vi "Go UP (Loaded).vi"(6 "Skip Loading?":bool, 7 "Model Name":T2, 8 "Error In":errorcluster, 9 "Intialize?":bool=TRUE, 10 "Inputs":T3) -> (0 "error out":errorcluster, 1 "Completed":bool, 3 "Results":T1, 4 "Status":cluster{"Status":string, "Elapsed Time":dbl}, 5 "Graph":dbl[][](array[numeric]))   [LabVIEW 2017]
doc: "Changelog:\n\n------------\nv0.1:\n- Bypass sensor 1 for all front\n\nv0.1:\n- Start Travel time taken from when the start moving command is given (previous state)\n- Total travel time is taken until the movement is stopped"
uses:
  controls/All Inputs.ctl
  controls/SACB DI.ctl
  controls/Model Name.ctl
  controls/Go UP (Loaded).ctl
  controls/FGV DO.ctl
panel:
  in  "Stall Time":u32=200
  out "Waveform Graph":dbl[][](graph)
  in  "Delay (for Rest)":u32=500
  in  "Timeout (ms)":u32=15000
  # "Inputs"
  # "Variables"
  # "Outputs"
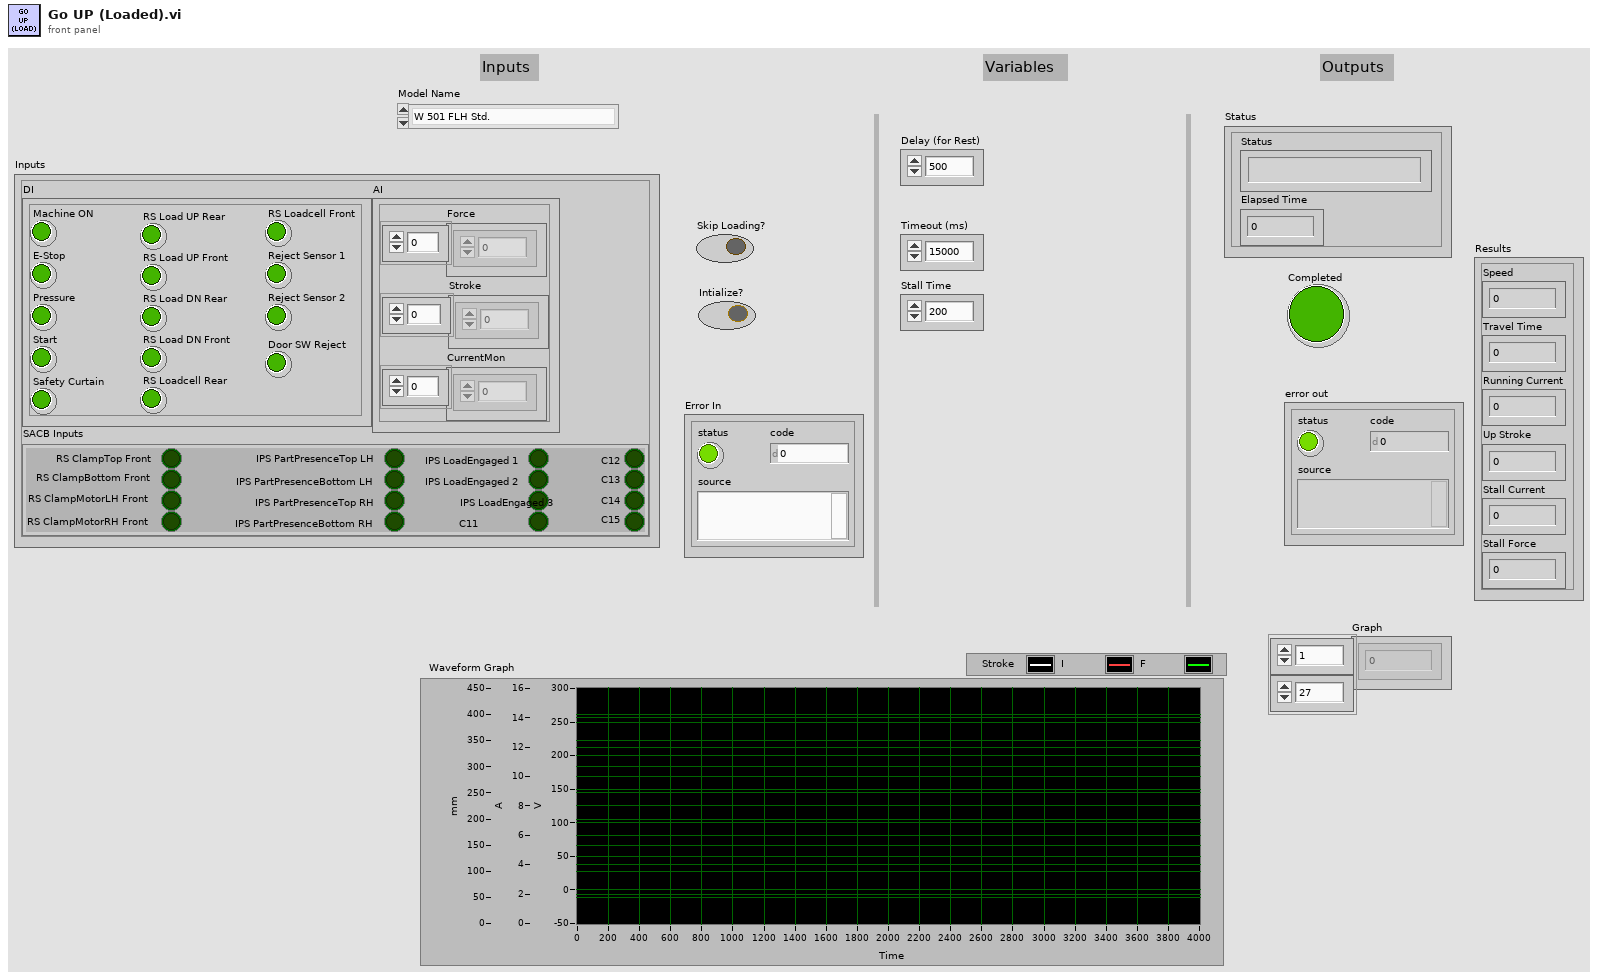
[diagram p1: front panel]
types:
  T1 = cluster{"Speed":dbl, "Travel Time":dbl, "Running Current":dbl, "Up Stroke":dbl, "Stall Current":dbl, "Stall Force":dbl}
  T2 = typedef "Model Name.ctl" = enum16{"W 501 FLH Std.", "W 501 FRH Std.", "W 601 FR RH Std", "W 601 FR LH Std", "W 601 RR RH Std", "W 601 RR LH Std", "W 601 FR RH AP", "W 601 FR LH AP", "W 601 RR RH AP", "W 601 RR LH AP"}
  T3 = typedef "All Inputs.ctl" = cluster{"DI":cluster{"Machine ON":bool, "E-Stop":bool, "Pressure":bool, "Start":bool, "Safety Curtain":bool, "RS Load UP Rear":bool, "RS Load UP Front":bool, "RS Load DN Rear":bool, "RS Load DN Front":bool, "RS Loadcell Rear":bool, "RS Loadcell Front":bool, "Reject Sensor 1":bool, "Reject Sensor 2":bool, "Door SW Reject":bool}, "AI":cluster{"Force":dbl[], "Stroke":dbl[], "CurrentMon":dbl[]}, "SACB Inputs":T4}
  T4 = typedef "SACB DI.ctl" = cluster{"RS ClampTop Front":bool, "RS ClampBottom Front":bool, "RS ClampMotorLH Front":bool, "RS ClampMotorRH Front":bool, "IPS PartPresenceTop LH":bool, "IPS PartPresenceBottom LH":bool, "IPS PartPresenceTop RH":bool, "IPS PartPresenceBottom RH":bool, "IPS LoadEngaged 1":bool, "IPS LoadEngaged 2":bool, "IPS LoadEngaged 3":bool, "C11":bool, "C12":bool, "C13":bool, "C14":bool, "C15":bool}
  T5 = typedef "Go UP (Loaded).ctl" = enum16{"Initialize", "Load UP Enable", "Check Bottom Position", "Go UP", "Wait for Stall", "Turn Off Supply", "Wait for Rest", "Done", "Error"}
  T6 = typedef "FGV DO.ctl" = enum16{"Initialize", "Start Task", "Clamping", "Load CYL", "Contactors", "Loadcell CYL", "BSL", "Read DO", "Clear Tasks", "Clear Task"}
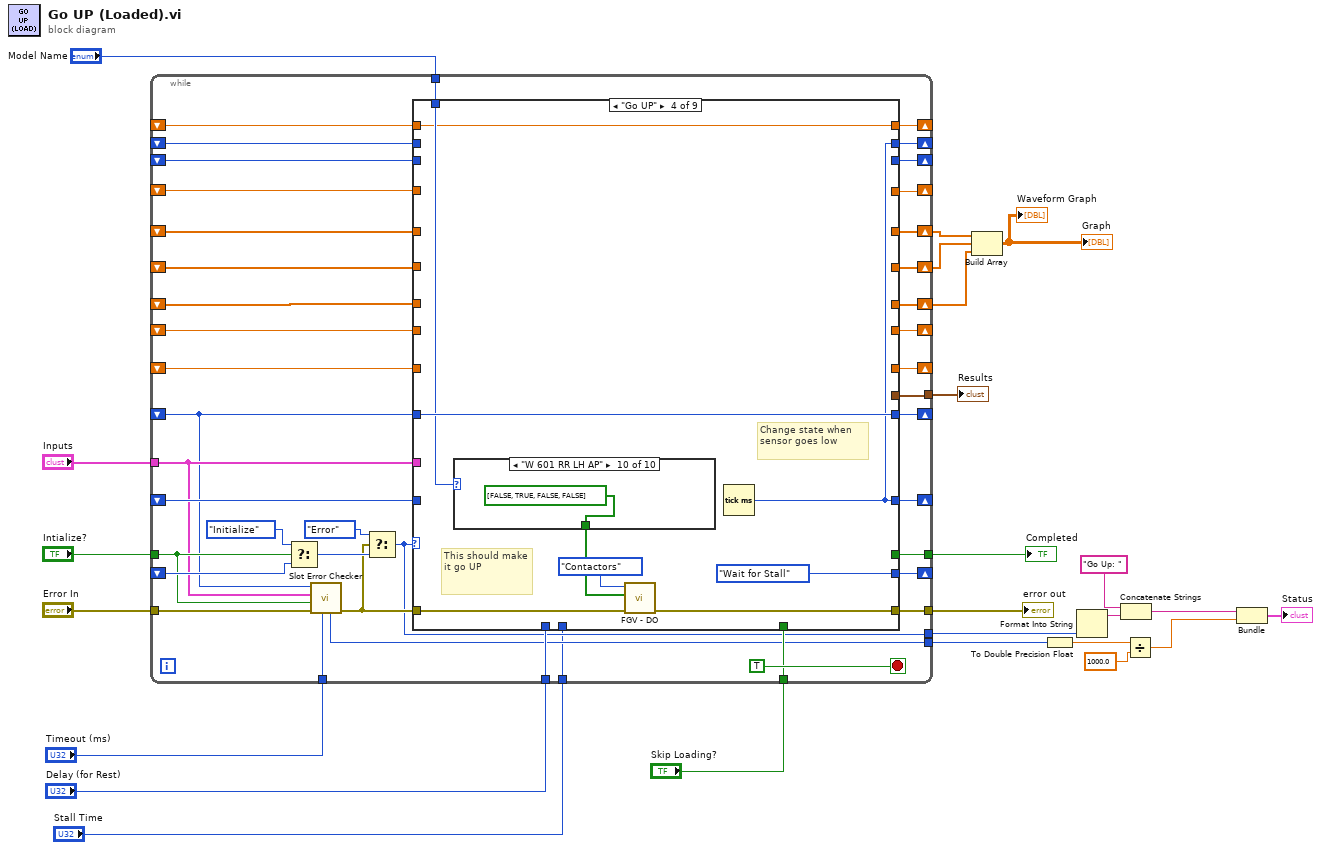
[diagram p0: block diagram]
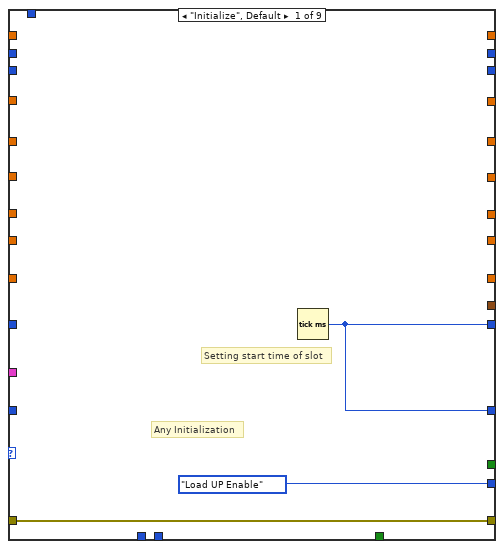
[diagram p2: hidden frame]
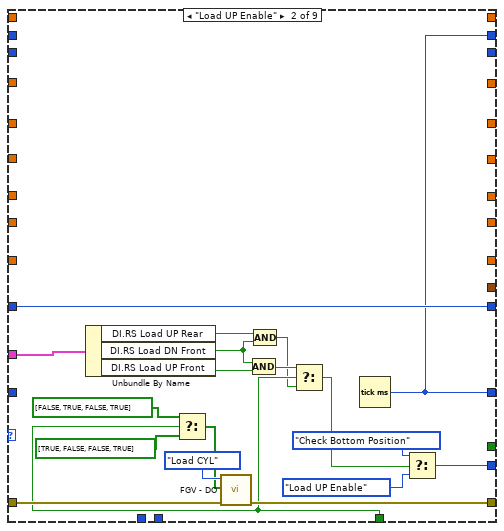
[diagram p3: hidden frame]
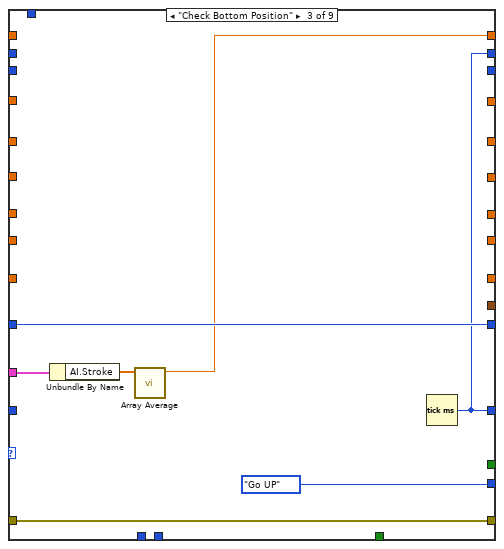
[diagram p4: hidden frame]
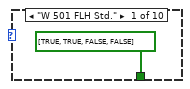
[diagram p5: hidden frame]
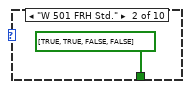
[diagram p6: hidden frame]
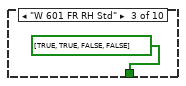
[diagram p7: hidden frame]
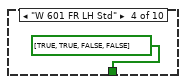
[diagram p8: hidden frame]
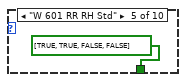
[diagram p9: hidden frame]
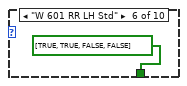
[diagram p10: hidden frame]
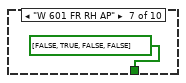
[diagram p11: hidden frame]
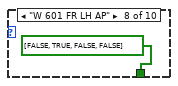
[diagram p12: hidden frame]
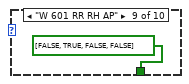
[diagram p13: hidden frame]
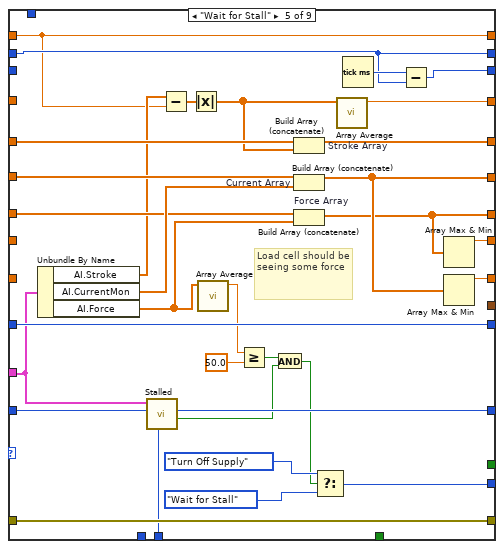
[diagram p14: hidden frame]
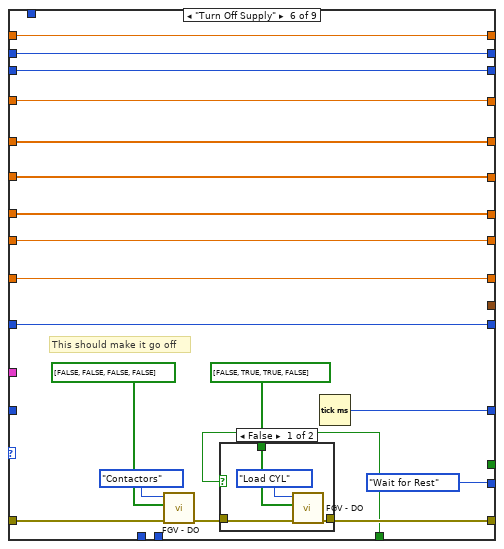
[diagram p15: hidden frame]
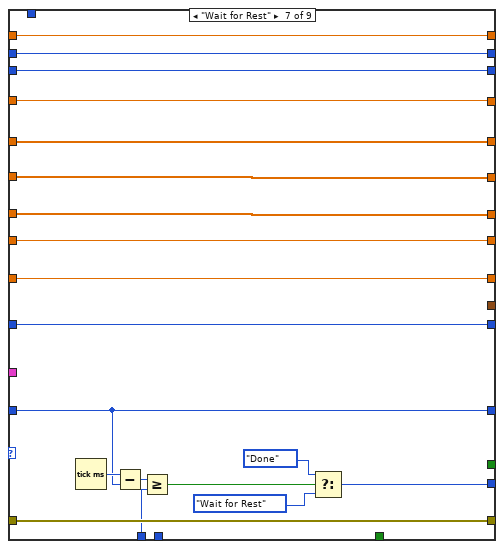
[diagram p17: hidden frame]
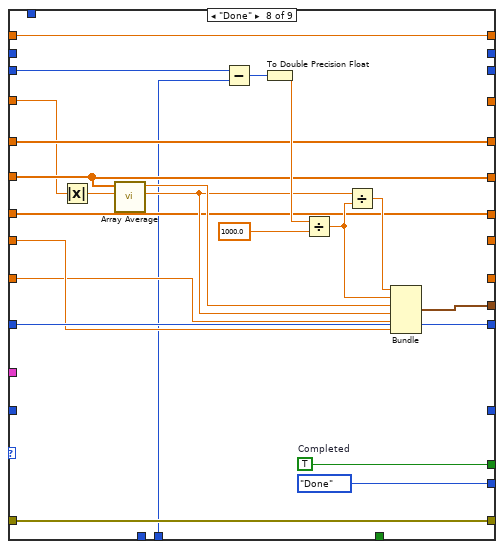
[diagram p18: hidden frame]
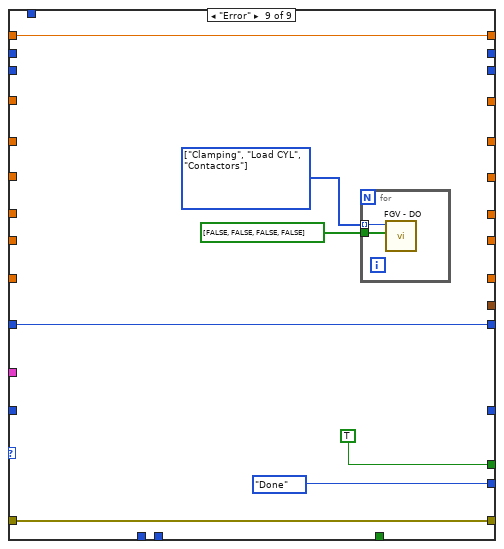
[diagram p19: hidden frame]
diagram:
  n1 = while {
    tunnel: "Intialize?" -> [w56]
    shift-right: [w63] -> _
    shift-left: _ -> [w65]
    shift-right: [w62] -> _
    shift-left: _ -> [w61]
    tunnel: "Error In" -> [w57]
    tunnel: [w60] -> w24
    tunnel: [w59] -> w23
    tunnel: "Inputs" -> [w55]
    shift-right: [w58] -> _
    shift-left: _ -> [w54]
    tunnel: "Delay (for Rest)" -> [w50]
    tunnel: "Timeout (ms)" -> [w49]
    tunnel: "Model Name" -> [w48]
    shift-right: [w47] -> _
    shift-left: _ -> [w46]
    shift-right: [w45] -> w5
    shift-left: _ -> [w44]
    shift-right: [w43] -> _
    shift-left: _ -> [w42]
    tunnel: [w41] -> w16
    tunnel: "Skip Loading?" -> [w40]
    shift-right: [w39] -> _
    shift-left: _ -> [w38]
    tunnel: [w37] -> w7
    tunnel: [w36] -> w6
    shift-right: [w35] -> _
    shift-left: _ -> [w34]
    shift-right: [w33] -> w4
    shift-left: _ -> [w32]
    shift-right: [w31] -> w2
    shift-left: _ -> [w30]
    shift-right: [w29] -> _
    shift-left: _ -> [w28]
    shift-right: [w27] -> _
    shift-left: _ -> [w26]
    tunnel: "Stall Time" -> [w25]
    stop <- TRUE stop-if-true
    n2 = Select(t=Go_UP_(Loaded)."Initialize", s=w56, f=w65) -> (s? t:f=w53:T5)
    n3 = call "Slot Error Checker.vi"("Timeout (ms)"=w49, "error in (no error)"=w57, "Intialize?"=w56, "Inputs"=w55, "start time"=w54) -> ("error out"=w52:errorcluster, "Slot Time"=w37:u32)  [unwired: 4 in, 1 out]
    n4 = Select(t=Go_UP_(Loaded)."Error", s=w52, f=w53) -> (s? t:f=w36:T5)
    n5 = case shown="\"Go UP\"" w36 {
      tunnel: [Go_UP_(Loaded)."Load UP Enable" w84 Go_UP_(Loaded)."Go UP" Go_UP_(Loaded)."Wait for Stall" w141 Go_UP_(Loaded)."Wait for Rest" w186 Go_UP_(Loaded)."Done" Go_UP_(Loaded)."Done"] -> w63
      tunnel: [w67 w80 w89 w96 w131 w162 w188 _ _] -> w62
      tunnel: w61 -> [_ _ _ _ w144 _ w188 _ _]
      tunnel: w52 -> [w68 w88 w94 w104 w145 w165 w184 w209 w217]
      tunnel: [w68 w87 w94 w103 w145 w149 w184 w209 w217] -> w60
      tunnel: [_ _ _ _ _ _ _ w208 TRUE ("Completed")] -> w59
      tunnel: w55 -> [_ w85 w91 _ w140 _ _ _ _]
      tunnel: [w67 w86 w95 w101 w146 w161 w181 w207 w214] -> w58
      tunnel: w54 -> [_ w86 w95 w101 w146 w161 w181 w207 w214]
      tunnel: w50 -> [_ _ _ _ _ _ w180 _ _]
      tunnel: w48 -> [_ _ _ w100 _ _ _ _ _]
      tunnel: [_ w80 w89 w96 w130 w158 w177 _ _] -> w47
      tunnel: w46 -> [_ _ _ _ w130 w158 w177 _ _]
      tunnel: [_ _ _ _ w132 w160 w179 w199 _] -> w45
      tunnel: w44 -> [_ _ _ _ w123 w160 w179 w199 _]
      tunnel: [_ _ _ _ w133 w159 w178 _ _] -> w43
      tunnel: w42 -> [_ _ _ _ _ w159 w178 w193 _]
      tunnel: [_ _ _ _ _ _ _ w201 _] -> w41
      tunnel: w40 -> [_ w73 _ _ _ w147 _ _ _]
      tunnel: [_ _ _ _ w138 w157 w176 _ _] -> w39
      tunnel: w38 -> [_ _ _ _ _ w157 w176 w195 _]
      tunnel: [_ _ w90 w99 w116 w156 w175 w196 w213] -> w35
      tunnel: w34 -> [_ _ _ w99 w116 w156 w175 w196 w213]
      tunnel: [_ _ _ _ w136 w154 w172 w198 _] -> w33
      tunnel: w32 -> [_ _ _ _ w122 w154 w172 w198 _]
      tunnel: [_ _ _ _ w135 w155 w173 w194 _] -> w31
      tunnel: w30 -> [_ _ _ _ w121 w155 w173 w194 _]
      tunnel: [_ _ _ _ w134 w151 w171 _ _] -> w29
      tunnel: w28 -> [_ _ _ _ _ w151 w171 w200 _]
      tunnel: [_ _ _ _ w120 w153 w174 _ _] -> w27
      tunnel: w26 -> [_ _ _ _ _ w153 w174 w190 _]
      tunnel: w25 -> [_ _ _ _ w119 _ _ w191 _]
      frame "Initialize", Default {
        # "Setting start time of slot"
        # "Any Initialization"
        n6 = Tick Count (ms)() -> (millisecond timer value=w67:u32)
      }
      frame "Load UP Enable" {
        n7 = Unbundle By Name(w85) -> ("DI.RS Load UP Rear"=w81:bool, "DI.RS Load DN Front"=w75:bool, "DI.RS Load UP Front"=w74:bool)
        n8 = Select(t=bool[] [FALSE, TRUE, FALSE, TRUE] ("Digital Outs"), s=w73, f=bool[] [TRUE, FALSE, FALSE, TRUE] ("Digital Outs")) -> (s? t:f=w77:bool[])
        n9 = call "FGV - DO.vi"("error in"=w88, "Digital Outs"=w77, "State"=FGV_DO."Load CYL") -> ("error out"=w87:errorcluster)  [unwired: 7 in, 1 out]
        n10 = Compound Arithmetic op=AND(w75, w74) -> (w71:bool)
        n11 = Compound Arithmetic op=AND(w81, w75) -> (w70:bool)
        n12 = Select(t=w71, s=w73, f=w70) -> (s? t:f=w72:bool)
        n13 = Tick Count (ms)() -> (millisecond timer value=w80:u32)
        n14 = Select(t=Go_UP_(Loaded)."Check Bottom Position", s=w72, f=Go_UP_(Loaded)."Load UP Enable") -> (s? t:f=w84:T5)
      }
      frame "Check Bottom Position" {
        n15 = Unbundle By Name(w91) -> ("AI.Stroke"=w92:dbl[])
        n16 = call "Array Average.vi"("data"=w92) -> ("Numeric"=w90:dbl)  [unwired: 10 in]
        n17 = Tick Count (ms)() -> (millisecond timer value=w89:u32)
      }
      frame "Go UP" {
        # "Change state when sensor goes low"
        # "This should make it go UP"
        n18 = case shown="\"W 601 RR LH AP\"" w100 {
          tunnel: [bool[] [TRUE, TRUE, FALSE, FALSE] ("Digital Outs") bool[] [TRUE, TRUE, FALSE, FALSE] ("Digital Outs") bool[] [TRUE, TRUE, FALSE, FALSE] ("Digital Outs") bool[] [TRUE, TRUE, FALSE, FALSE] ("Digital Outs") bool[] [TRUE, TRUE, FALSE, FALSE] ("Digital Outs") bool[] [TRUE, TRUE, FALSE, FALSE] ("Digital Outs") bool[] [FALSE, TRUE, FALSE, FALSE] ("Digital Outs") bool[] [FALSE, TRUE, FALSE, FALSE] ("Digital Outs") bool[] [FALSE, TRUE, FALSE, FALSE] ("Digital Outs") bool[] [FALSE, TRUE, FALSE, FALSE] ("Digital Outs")] -> w102
          frame "W 501 FLH Std." {
          }
          frame "W 501 FRH Std." {
          }
          frame "W 601 FR RH Std" {
          }
          frame "W 601 FR LH Std" {
          }
          frame "W 601 RR RH Std" {
          }
          frame "W 601 RR LH Std" {
          }
          frame "W 601 FR RH AP" {
          }
          frame "W 601 FR LH AP" {
          }
          frame "W 601 RR RH AP" {
          }
          frame "W 601 RR LH AP" {
          }
        }
        n19 = call "FGV - DO.vi"("error in"=w104, "Digital Outs"=w102, "State"=FGV_DO."Contactors") -> ("error out"=w103:errorcluster)  [unwired: 7 in, 1 out]
        n20 = Tick Count (ms)() -> (millisecond timer value=w96:u32)
      }
      frame "Wait for Stall" {
        # "Load cell should be seeing some force"
        n21 = Unbundle By Name(w140) -> ("AI.Stroke"=w118:dbl[], "AI.CurrentMon"=w137:dbl[], "AI.Force"=w125:dbl[])
        n22 = call "Stalled.vi"("Stall Time (ms)"=w119, "millisecond timer value in"=w144, "Inputs"=w140) -> ("Stalled"=w127:bool, "millisecond timer value out"=w131:u32)  [unwired: 7 in]
        n23 = Subtract(x=w118, y=w116) -> (x-y=w117:dbl[])
        n24 = Absolute Value(x=w117) -> (abs(x)=w115:dbl[])
        n25 = call "Array Average.vi"("data"=w125) -> ("Numeric"=w124:dbl)  [unwired: 10 in]
        n26 = Greater Or Equal?(x=w124, y=50.0) -> (x >= y?=w128:bool)
        n27 = And(x=w128, y=w127) -> (x .and. y?=w126:bool)
        n28 = Build Array (concatenate) "Stroke Array"(w123, w115) -> (w132:dbl[])
        n29 = Build Array (concatenate) "Current Array"(w122, w137) -> (w136:dbl[])
        n30 = Build Array (concatenate) "Force Array"(w121, w125) -> (w135:dbl[])
        n31 = Select(t=Go_UP_(Loaded)."Turn Off Supply", s=w126, f=Go_UP_(Loaded)."Wait for Stall") -> (s? t:f=w141:T5)
        n32 = call "Array Average.vi"("data"=w115) -> ("Numeric"=w120:dbl)  [unwired: 10 in]
        n33 = Tick Count (ms)() -> (millisecond timer value=w139:u32)
        n34 = Subtract(x=w139, y=w130) -> (x-y=w133:u32)
        n35 = Array Max & Min(array=w135) -> (max value=w134:dbl)  [unwired: 3 out]
        n36 = Array Max & Min(array=w136) -> (max value=w138:dbl)  [unwired: 3 out]
      }
      frame "Turn Off Supply" {
        # "This should make it go off"
        n37 = call "FGV - DO.vi"("error in"=w165, "Digital Outs"=bool[] [FALSE, FALSE, FALSE, FALSE], "State"=FGV_DO."Contactors") -> ("error out"=w150:errorcluster)  [unwired: 7 in, 1 out]
        n38 = case shown="False" w147 {
          tunnel: w150 -> [w168 w170]
          tunnel: [w167 w170] -> w149
          tunnel: bool[] [FALSE, TRUE, TRUE, FALSE] ("Digital Outs") -> [w166 _]
          frame False {
            n39 = call "FGV - DO.vi"("error in"=w168, "Digital Outs"=w166, "State"=FGV_DO."Load CYL") -> ("error out"=w167:errorcluster)  [unwired: 7 in, 1 out]
          }
          frame True {
          }
        }
        n40 = Tick Count (ms)() -> (millisecond timer value=w162:u32)
      }
      frame "Wait for Rest" {
        n41 = Tick Count (ms)() -> (millisecond timer value=w189:u32)
        n42 = Subtract(x=w189, y=w188) -> (x-y=w187:u32)
        n43 = Greater Or Equal?(x=w187, y=w180) -> (x >= y?=w185:bool)
        n44 = Select(t=Go_UP_(Loaded)."Done", s=w185, f=Go_UP_(Loaded)."Wait for Rest") -> (s? t:f=w186:T5)
      }
      frame "Done" {
        w208 = TRUE  # Completed
        n45 = Absolute Value(x=w190) -> (abs(x)=w197:dbl)
        n46 = call "Array Average.vi"("data"=w198) -> ("Numeric"=w202:dbl)  [unwired: 10 in]
        n47 = Subtract(x=w193, y=w191) -> (x-y=w192:u32)
        n48 = To Double Precision Float(number=w192) -> (double precision float=w205:dbl)
        n49 = Divide(x=w205, y=1000.0) -> (x/y=w203:dbl)
        n50 = Divide(x=w197, y=w203) -> (x/y=w204:dbl)
        n51 = Bundle(w204, w203, "Numeric"=w202, w197, w195, w200) -> (w201:cluster{dbl, dbl, "Numeric":dbl, dbl, dbl, dbl})  [unwired: 1 in]
      }
      frame "Error" {
        w211 = T6[] [enum."Clamping", enum."Load CYL", enum."Contactors"] items=["Initialize", "Start Task", "Clamping", "Load CYL", "Contactors", "Loadcell CYL", "BSL", "Read DO", "Clear Tasks", "Clear Task"]
        n52 = for {
          tunnel: w211 -> [w219] mode=indexing
          tunnel: bool[] [FALSE, FALSE, FALSE, FALSE] ("Digital Outs") -> [w218]
          n53 = call "FGV - DO.vi"("Digital Outs"=w218, "State"=w219) -> ()  [unwired: 8 in, 2 out]
        }
      }
    }
  }
  "error out" <- w24
  "Completed" <- w23
  "Results" <- w16
  n54 = Build Array(w5, w4, w2) -> (→"Graph" →"Waveform Graph":dbl[][])
  n55 = To Double Precision Float(number=w7) -> (double precision float=w12:dbl)
  n56 = Format Into String(w6) -> (resulting string=w14:string)  [unwired: 3 in, 1 out]
  n57 = Concatenate Strings("Go Up: ", w14) -> (w10:string)
  n58 = Divide(x=w12, y=1000.0) -> (x/y=w9:dbl)
  n59 = Bundle(w10, w9) -> (→"Status":cluster{string, dbl})  [unwired: 1 in]
